vi "split_state_and_argument.vi"(10 "String":string) -> (1 "Arguments":string, 3 "State":string)   [LabVIEW 2015]
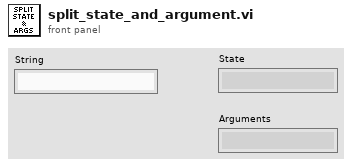
[diagram p1: front panel]
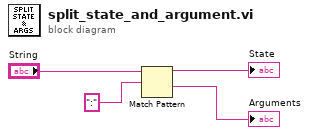
[diagram p0: block diagram]
diagram:
  n1 = Match Pattern(string="String", regular expression=":") -> (before substring=→"State":string, after substring=→"Arguments":string)  [unwired: 1 in, 2 out]
